vi "generator1.vi"() -> ()   [LabVIEW 2025]
panel:
  out "Waveform Graph":dbl[](graph)
  in  "phase":dbl
  in  "freq":dbl
  in  "Amp":dbl
  out "Waveform Chart":dbl(graph)
  in  "stop":bool
  in  "Sygnal":T1(ring)
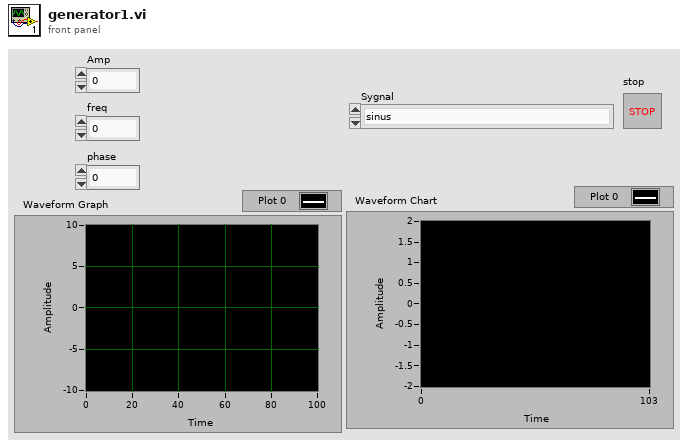
[diagram p1: front panel]
types:
  T1 = enum16{"sinus", "prostokat", "pila", "trojkat", "rozklad losowy", "rozklad normalny"}
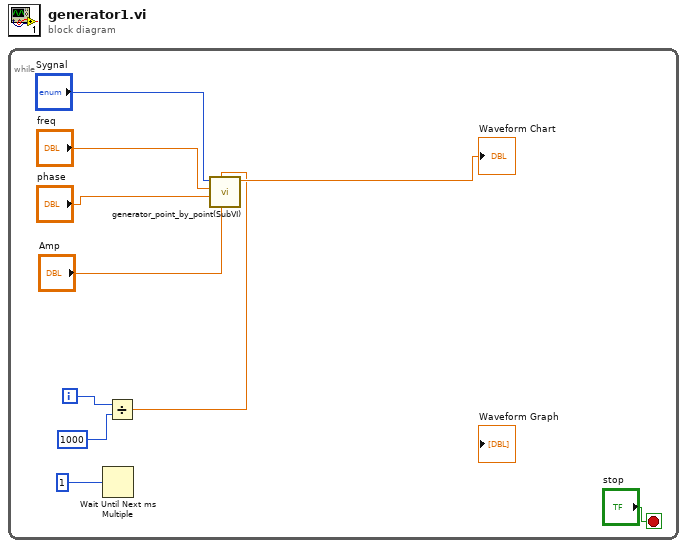
[diagram p0: block diagram]
diagram:
  n1 = while {
    i -> [w3]
    stop <- "stop" stop-if-true
    n2 = Wait Until Next ms Multiple(millisecond multiple=1) -> ()  [unwired: 1 out]
    n3 = Divide(x=w3, y=1000) -> (x/y=w1:dbl)
    n4 = call "generator_point_by_point(SubVI).vi"("Amp"="Amp", "Numeric"=w1, "phase"="phase", "freq"="freq", "Sygnal"="Sygnal") -> ("Gaussian white noise"=→"Waveform Chart":dbl)  [unwired: 6 in]
  }
